vi "control difuso simo legoappaf.vi"() -> ()   [LabVIEW 2020]
uses:
  <vilib>/addons/Fuzzy Logic/FL Fuzzy Controller (SIMO).vi
  <vilib>/addons/Fuzzy Logic/NI_Fuzzy_Logic_API.lvlib
panel:
  out "Array":dbl[][](array[numeric])
  in  "file path":path
  out "distancia":dbl(slide) scale=0.0..100.0
  out "angulo":dbl(knob) scale=-25.0..25.0
  in  "Reset":bool
  out "Motor Izquierda":dbl(slide) scale=-100.0..100.0
  out "Motor Derecha":dbl(slide) scale=-100.0..100.0
  out "Plano de trabajo":picture
  in  "stop":bool
  # "Ceballos Conde Emanuel\n4MV6\nSistemas de visión artificial\n2022/1"
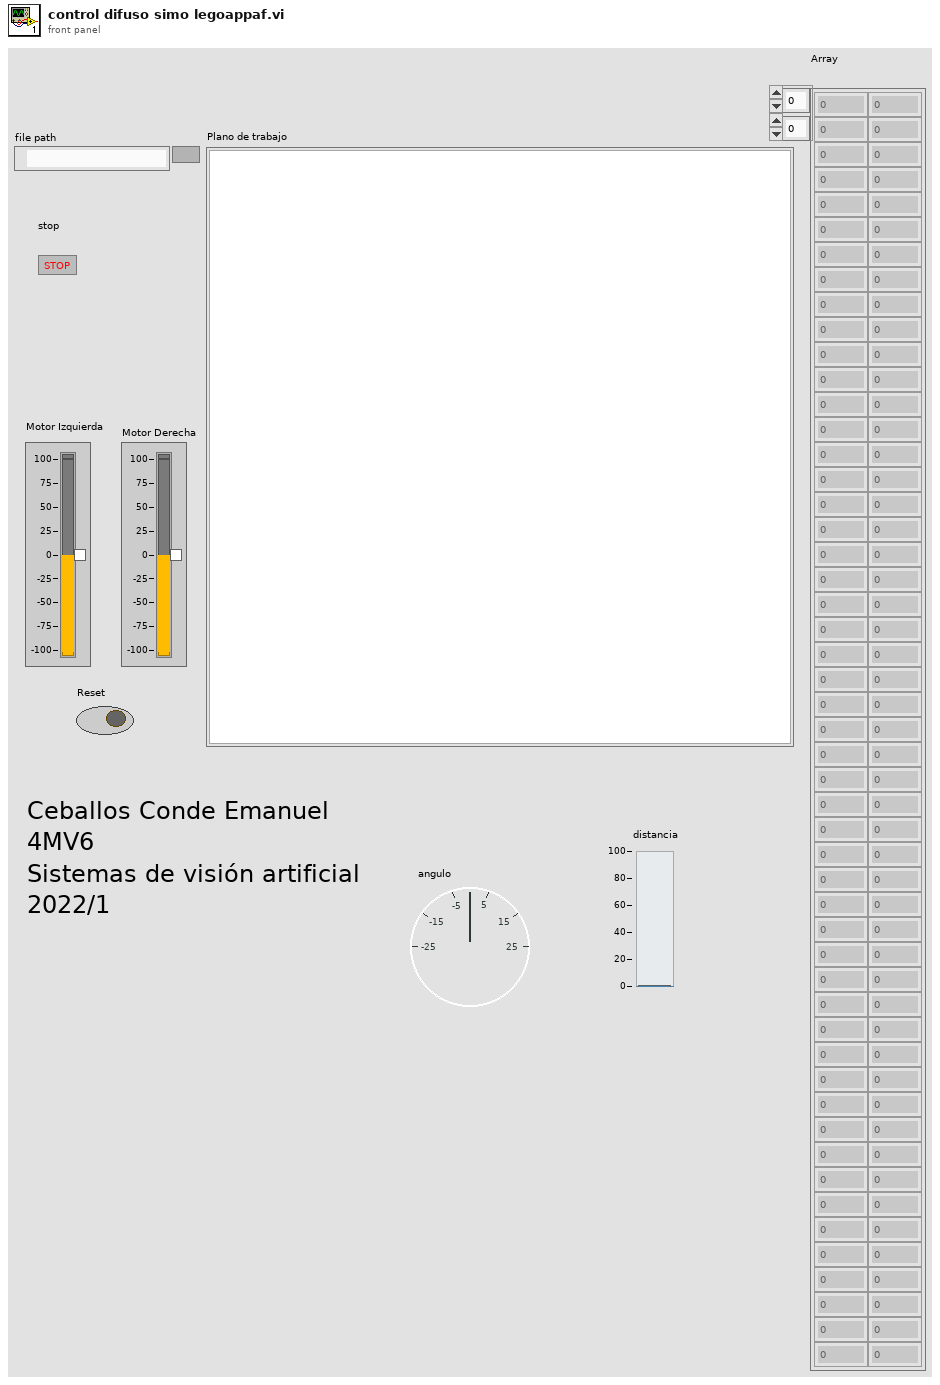
[diagram p1: front panel]
types:
  T1 = typedef "NI_Fuzzy_Logic_API.lvlib/FL System.ctl" = cluster{"input variables":T2[], "output variables":T2[], "rules":T5[], "defuzzification method":T11, "description":string, "user MF interpolating polynomials":T12[]}
  T2 = typedef "NI_Fuzzy_Logic_API.lvlib/FL Variable.ctl" = cluster{"name":string, "range":dbl[], "MFs":T3[]}
  T3 = typedef "NI_Fuzzy_Logic_API.lvlib/FL Membership Function.ctl" = cluster{"name":string, "shape":T4, "points":dbl[], "color":u32, "user-defined shape index":i32}
  T4 = typedef "NI_Fuzzy_Logic_API.lvlib/FL Membership Function Shape.ctl" = u16
  T5 = typedef "NI_Fuzzy_Logic_API.lvlib/FL Rule.ctl" = cluster{"antecedents":T6[], "antecedent connective":T8, "consequents":T9[], "consequent implication":T10, "degree of support":dbl}
  T6 = typedef "NI_Fuzzy_Logic_API.lvlib/FL Antecedent.ctl" = cluster{"Var Index":i32, "MF Index":i32, "Cond":T7}
  T7 = typedef "NI_Fuzzy_Logic_API.lvlib/FL Modifier.ctl" = u16
  T8 = typedef "NI_Fuzzy_Logic_API.lvlib/FL Antecedent Connective.ctl" = u16
  T9 = typedef "NI_Fuzzy_Logic_API.lvlib/FL Consequent.ctl" = cluster{"Var Index":i32, "MF Index":i32, "Cond":T7}
  T10 = typedef "NI_Fuzzy_Logic_API.lvlib/FL Consequent Implication.ctl" = u16
  T11 = typedef "NI_Fuzzy_Logic_API.lvlib/FL Defuzzification.ctl" = u16
  T12 = typedef "NI_Fuzzy_Logic_API.lvlib/FL Interpolating polynomials.ctl" = cluster{"X":dbl[], "Y":dbl[], "Y(x) coeff":dbl[][], "X(y) coeff":dbl[][], "Area(y) coeff":dbl[][], "coa_x(y) coeff":dbl[][]}
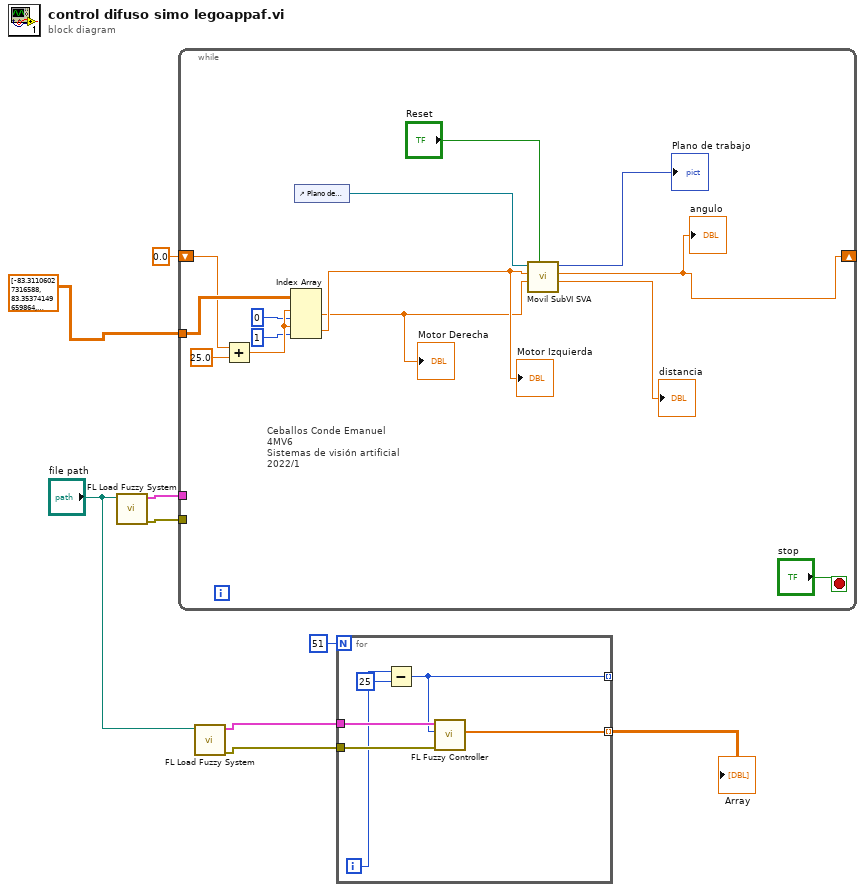
[diagram p0: block diagram]
diagram:
  n1 = call <vilib>:"FL Load Fuzzy System.vi"("file path"="file path") -> ("error out"=w8:errorcluster, "fuzzy system out"=w9:T1)  [unwired: 9 in]
  n2 = while {
    tunnel: w9 -> [_]
    tunnel: w8 -> [_]
    tunnel: dbl[][] [[-83.31106027316588, 83.35374149659864], [-83.31106027316588, 83.35374149659864], [-83.31106027316588, 83.35374149659864], [-83.31106027316588, 83.35374149659864], [-83.31106027316588, 83.35374149659864], [-83.31106027316588, 83.35374149659864], [-74.01277353631832, 74.03796024148275], [-68.07434564122147, 68.00511012645946], [-64.22359264049538, 64.26985448634075], [-61.85036028480257, 61.84544365353443], [-60.416548629446226, 60.397959183673485], [-58.83316612270298, 58.82380400694276], [-56.44469417107301, 56.37487347274782], [-53.29893444875278, 53.329179665034246], [-50.931657530132654, 50.91651613916596], [-49.98639455782313, 49.98301207275363], [-49.99485393171054, 49.980423000570134], [-49.98158448941816, 49.98654562449547], [-49.98418261482551, 49.960179193628676], [-49.974388698676286, 49.97300507504588], [-49.98639455782312, 50.00000000000001], [-46.36356473091168, 45.92783673469388], [-40.86322931096543, 40.40671843958822], [-35.49729206269503, 34.96882455720229], [-25.618693119655767, 25.142516804220207], [-0.2111189303307497, -0.2111189303307497], [25.142516804220207, -25.618693119655767], [34.96882455720229, -35.49729206269503], [40.40671843958822, -40.86322931096543], [45.92783673469388, -46.36356473091168], [50.00000000000001, -49.98639455782312], [49.97300507504588, -49.974388698676286], [49.960179193628676, -49.98418261482551], [49.98654562449547, -49.98158448941816], [49.980423000570134, -49.99485393171054], [49.98301207275363, -49.98639455782313], [50.91651613916596, -50.931657530132654], [53.329179665034246, -53.29893444875278], [56.37487347274782, -56.44469417107301], [58.82380400694276, -58.83316612270298], [60.397959183673485, -60.416548629446226], [61.84544365353443, -61.85036028480257], [64.26985448634075, -64.22359264049538], [68.00511012645946, -68.07434564122147], [74.03796024148275, -74.01277353631832], [83.35374149659864, -83.31106027316588], [83.35374149659864, -83.31106027316588], [83.35374149659864, -83.31106027316588], [83.35374149659864, -83.31106027316588], [83.35374149659864, -83.31106027316588], [83.35374149659864, -83.31106027316588]] ("Array") -> [w18]
    shift-right: [w16] -> _
    shift-left: 0.0 ("Angulo") -> [w15]
    stop <- "stop" stop-if-true
    # "Ceballos Conde Emanuel\n4MV6\nSistemas de visión artificial\n2022/1"
    n3 = Add(x=w15, y=25.0) -> (x+y=w14:dbl)
    n4 = Index Array(array=w18, index (row) #1=w14, index (col) #1=0 ("disabled index (col)"), index (row) #2=w14, index (col) #2=1 ("disabled index (col)")) -> (element #1=w10:dbl, element #2=w11:dbl)
    "Motor Derecha" <- w10
    "Motor Izquierda" <- w11
    n5 = control-ref of="Plano de trabajo"() -> (w21:refnum<vi>)
    n6 = call "Movil SubVI SVA.vi"("Reset"="Reset", "Motor Izquierda"=w10, "Motor Derecha"=w11, "Ref Plano"=w21) -> ("Distancia"=→"distancia":dbl, "Angulo"=w16:dbl, "Plano de trabajo"=→"Plano de trabajo":picture)  [unwired: 3 in, 2 out]
    "angulo" <- w16
  }
  n7 = call <vilib>:"FL Load Fuzzy System.vi"("file path"="file path") -> ("error out"=w6:errorcluster, "fuzzy system out"=w7:T1)  [unwired: 9 in]
  n8 = for {
    N: 51 -> [_]
    tunnel: w7 -> [w29]
    tunnel: w6 -> [w28]
    tunnel: [w24] -> _ mode=indexing
    tunnel: [w25] -> w4 mode=indexing
    i -> [w27]
    n9 = Subtract(x=w27, y=25) -> (x-y=w24:i32)
    n10 = call-poly <vilib>:"FL Fuzzy Controller.vi"("error in (no error)"=w28, "input value"=w24, "fuzzy system in"=w29) -> ("output values"=w25:dbl[])  [unwired: 4 in, 4 out]
  }
  "Array" <- w4
